vi "shooter control.vi"(0 "Back Shooter DevRef In":T1={"DeviceStatus"={"status"=FALSE, "code"=0, "source"=""}, "Type"=enum."PWM", "PWM"={"Digital Module"=enum."Digital Module 2", "PWM Channel"=enum."PWM 1", "DeadBand"={"Name"="", "maxPositivePwm"=0, "minPositivePwm"=0, "centerPwm"=0, "maxNegativePwm"=0, "minNegativePwm"=0, "angularRange"=0}}, "CAN"={"Device Number"=0, "Control Mode"=enum."Percent VBus", "Semaphore"=refnum, "Max Vout"=12.0}, "Invert"=FALSE, "TransformRef"=refnum, "InvTransformRef"=refnum}, 1 "Front Shooter DevRef In":T1={"DeviceStatus"={"status"=FALSE, "code"=0, "source"=""}, "Type"=enum."PWM", "PWM"={"Digital Module"=enum."Digital Module 2", "PWM Channel"=enum."PWM 1", "DeadBand"={"Name"="", "maxPositivePwm"=0, "minPositivePwm"=0, "centerPwm"=0, "maxNegativePwm"=0, "minNegativePwm"=0, "angularRange"=0}}, "CAN"={"Device Number"=0, "Control Mode"=enum."Percent VBus", "Semaphore"=refnum, "Max Vout"=12.0}, "Invert"=FALSE, "TransformRef"=refnum, "InvTransformRef"=refnum}, 5 "Closed Loop On/Off":bool, 7 "Power On/Off":bool, 9 "Joystick Throttle":dbl, 11 "Target Button":bool, 12 "PyramidButton":bool) -> (3 "Front Shooter DevRef Out":T1={"DeviceStatus"={"status"=FALSE, "code"=0, "source"=""}, "Type"=enum."PWM", "PWM"={"Digital Module"=enum."Digital Module 2", "PWM Channel"=enum."PWM 1", "DeadBand"={"Name"="", "maxPositivePwm"=0, "minPositivePwm"=0, "centerPwm"=0, "maxNegativePwm"=0, "minNegativePwm"=0, "angularRange"=0}}, "CAN"={"Device Number"=0, "Control Mode"=enum."Percent VBus", "Semaphore"=refnum, "Max Vout"=12.0}, "Invert"=FALSE, "TransformRef"=refnum, "InvTransformRef"=refnum}, 4 "Back Shooter DevRef Out":T1={"DeviceStatus"={"status"=FALSE, "code"=0, "source"=""}, "Type"=enum."PWM", "PWM"={"Digital Module"=enum."Digital Module 2", "PWM Channel"=enum."PWM 1", "DeadBand"={"Name"="", "maxPositivePwm"=0, "minPositivePwm"=0, "centerPwm"=0, "maxNegativePwm"=0, "minNegativePwm"=0, "angularRange"=0}}, "CAN"={"Device Number"=0, "Control Mode"=enum."Percent VBus", "Semaphore"=refnum, "Max Vout"=12.0}, "Invert"=FALSE, "TransformRef"=refnum, "InvTransformRef"=refnum}, 6 "FrontShooterOut":dbl, 8 "BackShooterOut":dbl)   [LabVIEW 2012]
uses:
  <vilib>/Rock Robotics/WPI/MotorControl/WPI_MotorControlDeviceRef.ctl
  <vilib>/Rock Robotics/SystemInterfaces/Typedef/FPGA_TypedefDigitalModule.ctl
  <vilib>/Rock Robotics/SystemInterfaces/DIO/FPGA_DIOPWMChannel.ctl
  <vilib>/Rock Robotics/WPI/PWM/WPI_PWMDeadband.ctl
  <vilib>/Rock Robotics/WPI/CAN/Jaguar/SubVIs/WPI_CANJaguar_ControlMode.ctl
  <vilib>/Rock Robotics/WPI/PWM/WPI_PWMTransform_ConPane.ctl
  <vilib>/Rock Robotics/WPI/CAN/Jaguar/SubVIs/WPI_CANJaguar_SpeedReference.ctl
  Robot Global Data.vi
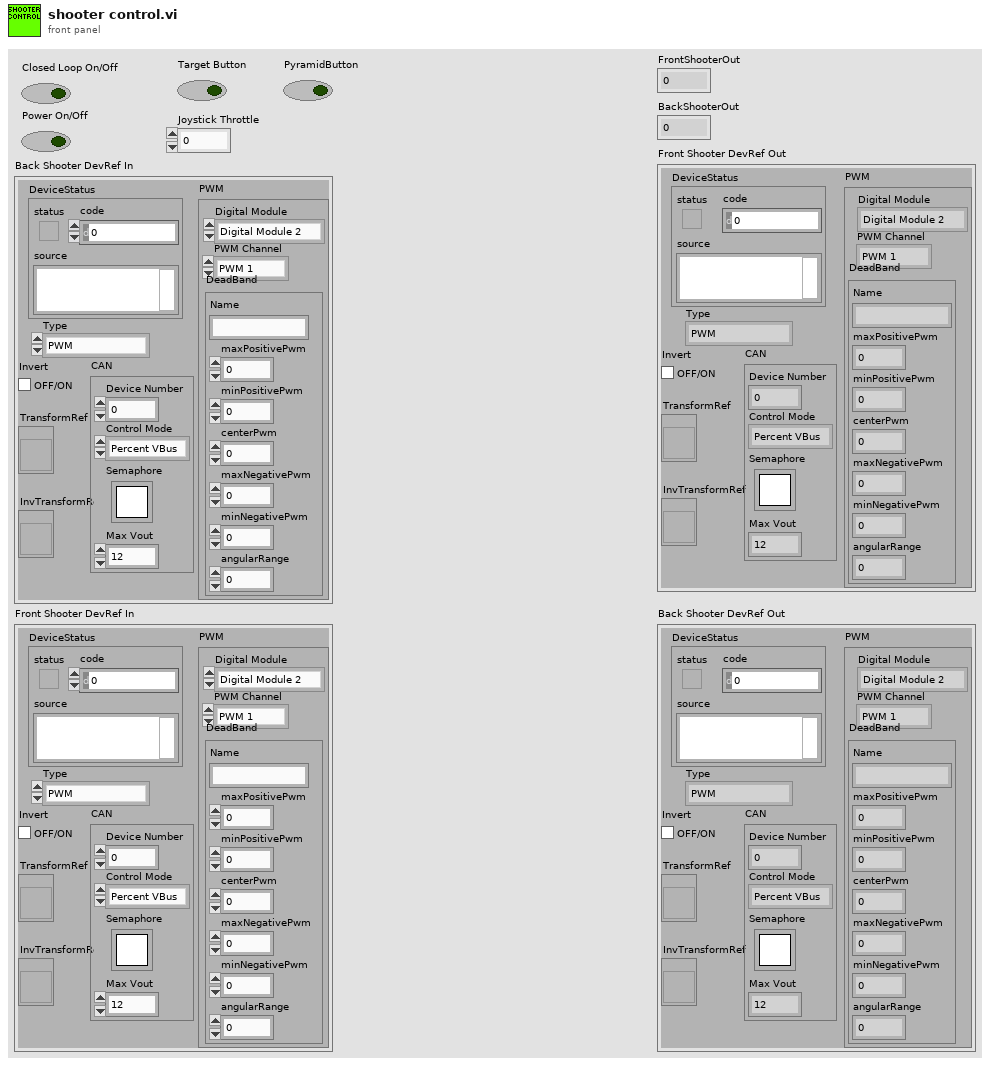
[diagram p1: front panel]
types:
  T1 = typedef "WPI_MotorControlDeviceRef.ctl" = cluster{"DeviceStatus":errorcluster, "Type":enum16{"PWM", "CAN"}, "PWM":cluster{"Digital Module":T2, "PWM Channel":T3, "DeadBand":T4}, "CAN":cluster{"Device Number":u8, "Control Mode":T5, "Semaphore":T6, "Max Vout":dbl}, "Invert":bool, "TransformRef":T7, "InvTransformRef":T7}
  T2 = typedef "FPGA_TypedefDigitalModule.ctl" = enum16{"Digital Module 1", "Digital Module 2"}
  T3 = typedef "FPGA_DIOPWMChannel.ctl" = enum8{"PWM 1", "PWM 2", "PWM 3", "PWM 4", "PWM 5", "PWM 6", "PWM 7", "PWM 8", "PWM 9", "PWM 10", "Invalid"}
  T4 = typedef "WPI_PWMDeadband.ctl" = cluster{"Name":string, "maxPositivePwm":i32, "minPositivePwm":i32, "centerPwm":i32, "maxNegativePwm":i32, "minNegativePwm":i32, "angularRange":u16}
  T5 = typedef "WPI_CANJaguar_ControlMode.ctl" = enum8{"Percent VBus", "Current", "Speed", "Position", "Voltage"}
  T6 = typedef "Semaphore RefNum" = refnum<k1>
  T7 = typedef "WPI_PWMTransform_ConPane.ctl" = refnum<vi>
  T8 = typedef "WPI_CANJaguar_SpeedReference.ctl" = u8
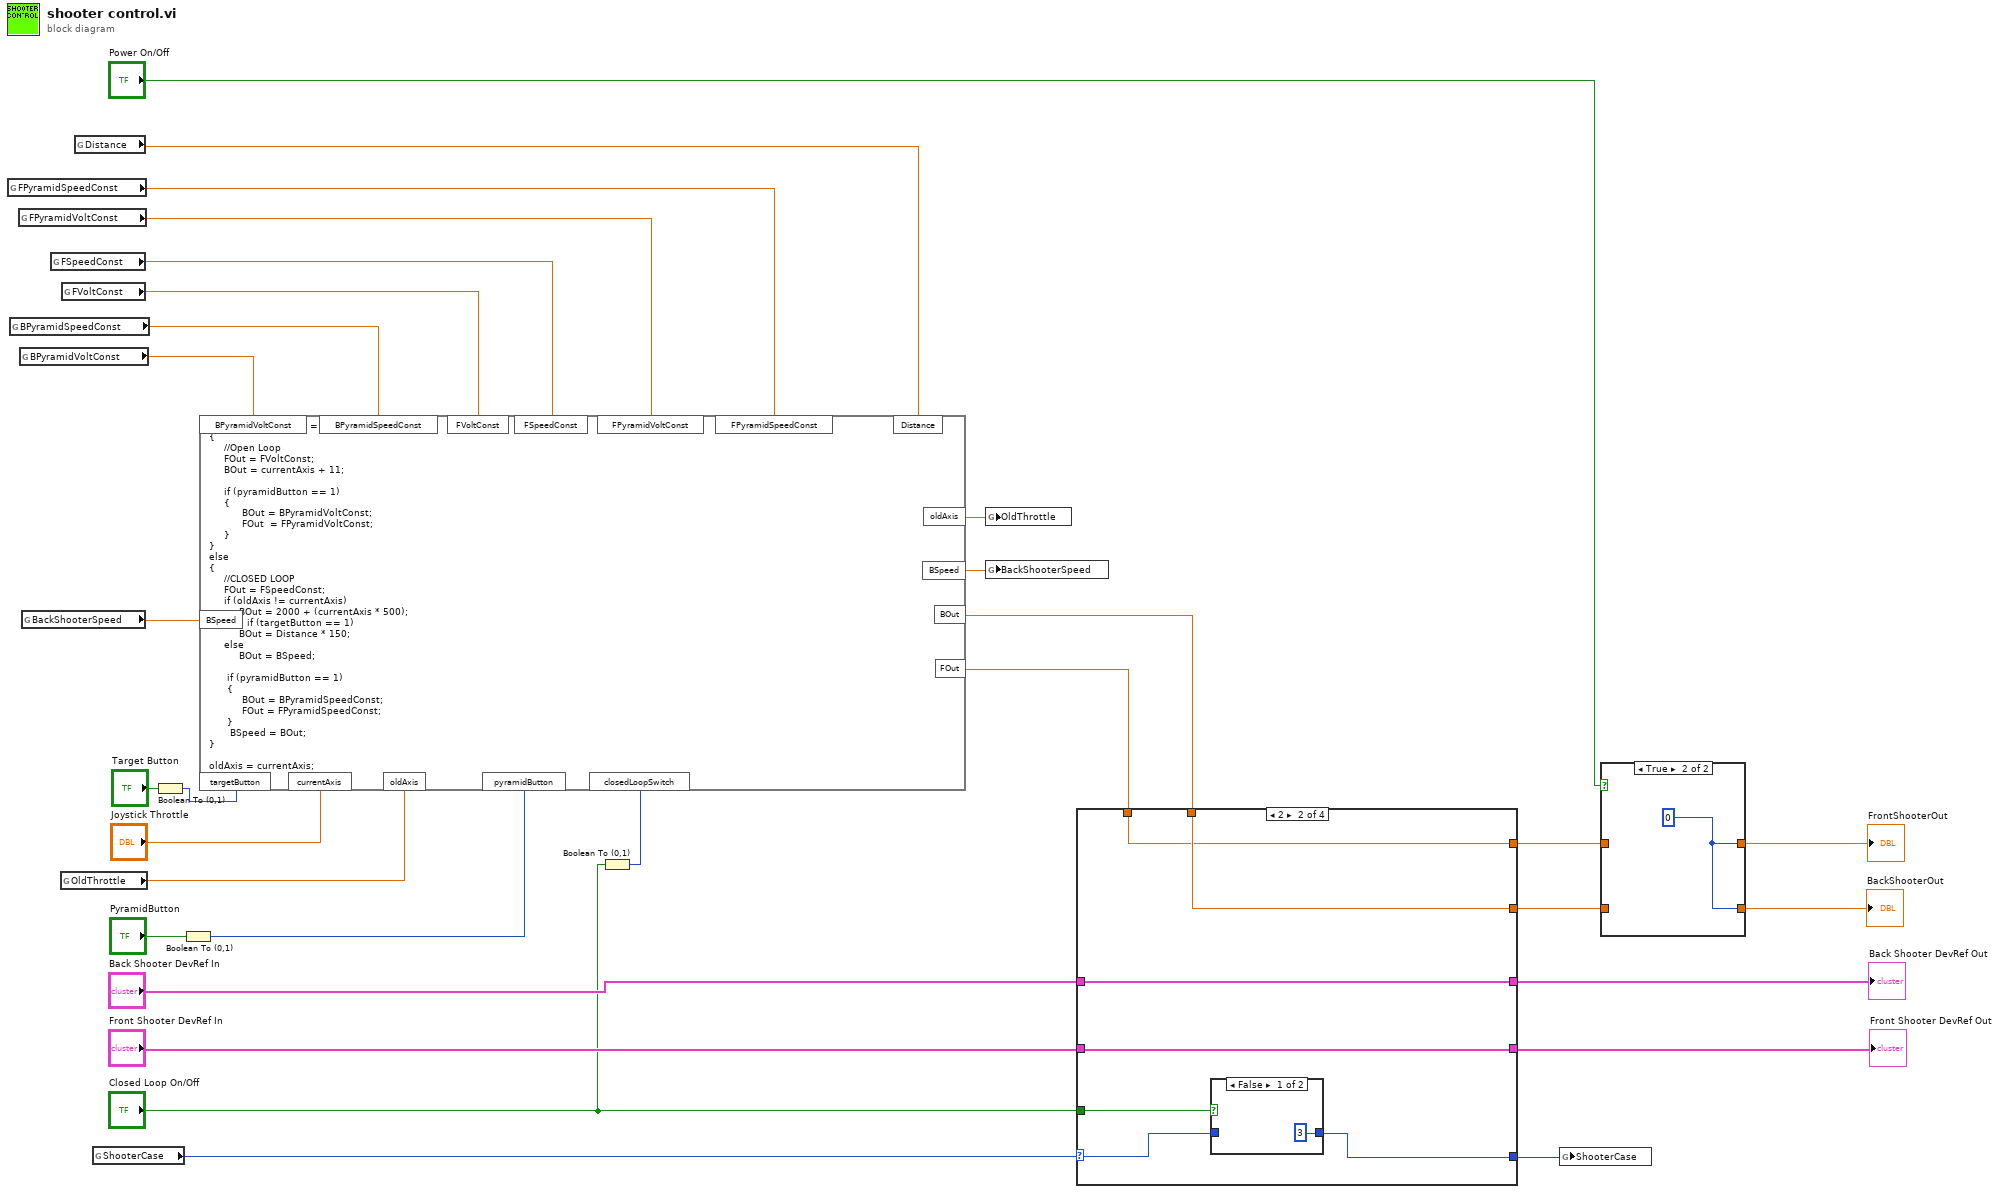
[diagram p0: block diagram]
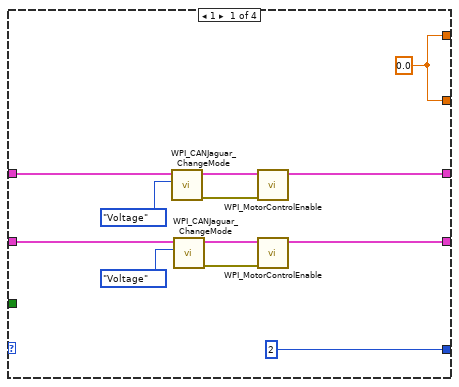
[diagram p3: hidden frame]
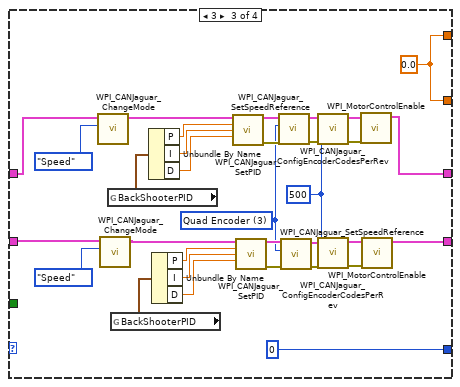
[diagram p5: hidden frame]
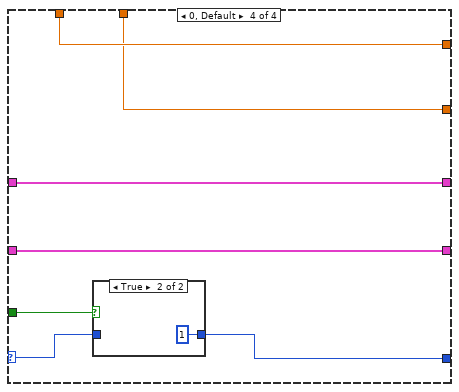
[diagram p6: hidden frame]
diagram:
  n1 = global read "Robot Global Data.vi" "FPyramidSpeedConst"() -> (w2:dbl)
  n2 = global read "Robot Global Data.vi" "BPyramidSpeedConst"() -> (w8:dbl)
  n3 = global read "Robot Global Data.vi" "FPyramidVoltConst"() -> (w3:dbl)
  n4 = global read "Robot Global Data.vi" "BPyramidVoltConst"() -> (w9:dbl)
  n5 = global read "Robot Global Data.vi" "BackShooterSpeed"() -> (w25:dbl)
  n6 = global read "Robot Global Data.vi" "FSpeedConst"() -> (w15:dbl)
  n7 = global read "Robot Global Data.vi" "OldThrottle"() -> (w5:dbl)
  n8 = global read "Robot Global Data.vi" "FVoltConst"() -> (w14:dbl)
  n9 = global read "Robot Global Data.vi" "Distance"() -> (w10:dbl)
  n10 = global read "Robot Global Data.vi" "ShooterCase"() -> (w27:i8)
  n11 = Boolean To (0,1)(Boolean="Target Button") -> (0, 1=w11:i16)
  n12 = Boolean To (0,1)(Boolean="PyramidButton") -> (0, 1=w6:i16)
  n13 = Boolean To (0,1)(Boolean="Closed Loop On/Off") -> (0, 1=w12:i16)
  n14 = formula code="if (closedLoopSwitch == 1)\n{\n     //Open Loop\n     FOut = FVoltConst;\n     BOut = currentAxis + 11;     \n\n     if (pyramidButton == 1)\n     {\n           BOut = BPyramidVoltConst;\n           FOut  = FPyramidVoltConst;\n     }                                                                    \n} \nelse\n{\n     //CLOSED LOOP\n     FOut = FSpeedConst;\n     if (oldAxis != currentAxis)\n          BOut = 2000 + (currentAxis * 500);\n     else if (targetButton == 1)\n          BOut = Distance * 150;\n     else\n          BOut = BSpeed;\n\n      if (pyramidButton == 1)\n      {\n           BOut = BPyramidSpeedConst;\n           FOut = FPyramidSpeedConst;\n      }\n       BSpeed = BOut;\n}\n\noldAxis = currentAxis;"("BSpeed"=w25, "closedLoopSwitch"=w12, "currentAxis"="Joystick Throttle", "FVoltConst"=w14, "FSpeedConst"=w15, "targetButton"=w11, "Distance"=w10, "BPyramidSpeedConst"=w8, "BPyramidVoltConst"=w9, "pyramidButton"=w6, "oldAxis"=w5, "FPyramidVoltConst"=w3, "FPyramidSpeedConst"=w2) -> ("BOut"=w18:dbl, "FOut"=w19:dbl, "oldAxis"=w4:dbl, "BSpeed"=w1:dbl)
  n15 = global write "Robot Global Data.vi" "OldThrottle"(w4) -> ()
  n16 = global write "Robot Global Data.vi" "BackShooterSpeed"(w1) -> ()
  n17 = case shown="2" w27 {
    selector: w27 -> [_ w47 _ w87]
    tunnel: [i8 2 ("ShooterCase") w46 i8 0 ("ShooterCase") w88] -> w26
    tunnel: "Back Shooter DevRef In" -> [w42 w50 w82 w91]
    tunnel: "Front Shooter DevRef In" -> [w41 w49 w81 w90]
    tunnel: [w34 w50 w54 w91] -> w29
    tunnel: [w33 w49 w55 w90] -> w28
    tunnel: "Closed Loop On/Off" -> [_ w48 _ w89]
    tunnel: w19 -> [_ w44 _ w86]
    tunnel: w18 -> [_ w45 _ w85]
    tunnel: [w32 w44 w53 w86] -> w17
    tunnel: [w32 w45 w53 w85] -> w16
    frame 1 {
      w32 = 0.0 ("FSpeed")
      n18 = call <vilib>:"WPI_CANJaguar_ChangeMode.vi"("Control Mode"=WPI_CANJaguar_ControlMode."Voltage", "CAN Jaguar Ref"=w42) -> ("error out"=w35:errorcluster, "CAN Jaguar Ref Out"=w36:T1)  [unwired: 8 in]
      n19 = call <vilib>:"WPI_CANJaguar_ChangeMode.vi"("Control Mode"=WPI_CANJaguar_ControlMode."Voltage", "CAN Jaguar Ref"=w41) -> ("error out"=w37:errorcluster, "CAN Jaguar Ref Out"=w38:T1)  [unwired: 8 in]
      n20 = call <vilib>:"WPI_MotorControlEnable.vi"("error in (no error)"=w35, "CAN Jaguar Ref"=w36) -> ("CAN Jaguar Ref Out"=w34:T1)  [unwired: 8 in, 1 out]
      n21 = call <vilib>:"WPI_MotorControlEnable.vi"("error in (no error)"=w37, "CAN Jaguar Ref"=w38) -> ("CAN Jaguar Ref Out"=w33:T1)  [unwired: 8 in, 1 out]
    }
    frame 2 {
      n22 = case shown="False" w48 {
        tunnel: [i8 3 ("ShooterCase") w52] -> w46
        tunnel: w47 -> [_ w52]
        frame False {
        }
        frame True {
        }
      }
    }
    frame 3 {
      w53 = 0.0 ("FSpeed")
      w60 = u16 500 ("Encoder Codes Per Rev")
      w65 = T8 3 items=["Encoder"=0, "Inv Encoder"=2, "Quad Encoder"=3, "None"=255] ("Speed Reference")
      n23 = call <vilib>:"WPI_CANJaguar_ChangeMode.vi"("Control Mode"=WPI_CANJaguar_ControlMode."Speed", "CAN Jaguar Ref"=w82) -> ("CAN Jaguar Ref Out"=w80:T1)  [unwired: 8 in, 1 out]
      n24 = call <vilib>:"WPI_CANJaguar_ChangeMode.vi"("Control Mode"=WPI_CANJaguar_ControlMode."Speed", "CAN Jaguar Ref"=w81) -> ("CAN Jaguar Ref Out"=w71:T1)  [unwired: 8 in, 1 out]
      n25 = global read "Robot Global Data.vi" "BackShooterPID"() -> (w79:cluster{"P":dbl, "I":dbl, "D":dbl})
      n26 = global read "Robot Global Data.vi" "BackShooterPID"() -> (w75:cluster{"P":dbl, "I":dbl, "D":dbl})
      n27 = Unbundle By Name(w79) -> ("P"=w78:dbl, "I"=w77:dbl, "D"=w76:dbl)
      n28 = Unbundle By Name(w75) -> ("P"=w74:dbl, "I"=w73:dbl, "D"=w72:dbl)
      n29 = call <vilib>:"WPI_CANJaguar_SetPID.vi"("CAN Jaguar Ref"=w80, "P"=w78, "I"=w77, "D"=w76) -> ("CAN Jaguar Ref Out"=w68:T1, "error out"=w69:errorcluster)  [unwired: 10 in]
      n30 = call <vilib>:"WPI_CANJaguar_SetPID.vi"("CAN Jaguar Ref"=w71, "P"=w74, "I"=w73, "D"=w72) -> ("CAN Jaguar Ref Out"=w67:T1, "error out"=w66:errorcluster)  [unwired: 10 in]
      n31 = call <vilib>:"WPI_CANJaguar_SetSpeedReference.vi"("error in (no error)"=w69, "Speed Reference"=w65, "CAN Jaguar Ref"=w68) -> ("error out"=w64:errorcluster, "CAN Jaguar Ref Out"=w63:T1)  [unwired: 7 in]
      n32 = call <vilib>:"WPI_CANJaguar_SetSpeedReference.vi"("error in (no error)"=w66, "Speed Reference"=w65, "CAN Jaguar Ref"=w67) -> ("error out"=w61:errorcluster, "CAN Jaguar Ref Out"=w62:T1)  [unwired: 7 in]
      n33 = call <vilib>:"WPI_CANJaguar_ConfigEncoderCodesPerRev.vi"("error in (no error)"=w64, "Encoder Codes Per Rev"=w60, "CAN Jaguar Ref"=w63) -> ("error out"=w59:errorcluster, "CAN Jaguar Ref Out"=w58:T1)  [unwired: 7 in]
      n34 = call <vilib>:"WPI_CANJaguar_ConfigEncoderCodesPerRev.vi"("error in (no error)"=w61, "Encoder Codes Per Rev"=w60, "CAN Jaguar Ref"=w62) -> ("error out"=w57:errorcluster, "CAN Jaguar Ref Out"=w56:T1)  [unwired: 7 in]
      n35 = call <vilib>:"WPI_MotorControlEnable.vi"("error in (no error)"=w59, "CAN Jaguar Ref"=w58) -> ("CAN Jaguar Ref Out"=w54:T1)  [unwired: 8 in, 1 out]
      n36 = call <vilib>:"WPI_MotorControlEnable.vi"("error in (no error)"=w57, "CAN Jaguar Ref"=w56) -> ("CAN Jaguar Ref Out"=w55:T1)  [unwired: 8 in, 1 out]
    }
    frame 0, Default {
      n37 = case shown="True" w89 {
        tunnel: [w92 i8 1 ("ShooterCase")] -> w88
        tunnel: w87 -> [w92 _]
        frame False {
        }
        frame True {
        }
      }
    }
  }
  "Front Shooter DevRef Out" <- w28
  "Back Shooter DevRef Out" <- w29
  n38 = global write "Robot Global Data.vi" "ShooterCase"(w26) -> ()
  n39 = case shown="True" "Power On/Off" {
    tunnel: [w95 w96] -> w23
    tunnel: [w94 w96] -> w22
    tunnel: w17 -> [w95 _]
    tunnel: w16 -> [w94 _]
    frame False {
    }
    frame True {
      w96 = 0
    }
  }
  "FrontShooterOut" <- w23
  "BackShooterOut" <- w22
